vi "VIE.Module.Queued Message Handler.dqClass_ObjectReferenceToQueue.vi"(1 "reference":T1) -> (21 "queue":refnum<queue>)   [LabVIEW 2010, in "VIE.Module.Queued Message Handler.QueuedMessageHandler.dqGOOPClass.lvlib"]
doc: "Converts a dqGOOP object refnum to a queue refnum"
uses:
  VIE.Module.Queued Message Handler.QueuedMessageHandler.dqGOOPClass.lvlib
  VIE.Module.Queued Message Handler.dqClass_ObjectData.ctl
  VIE.Module.Queued Message Handler.dqClass_ObjectReference.ctl
panel:
  in  "queue (default)":refnum<queue>
  # "Copyright (C) 2004 DataAct Incorporated"
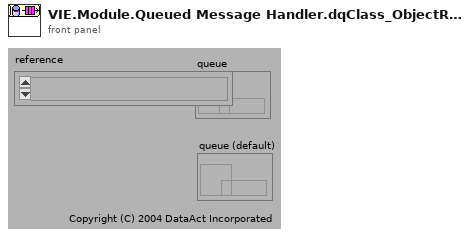
[diagram p1: front panel]
types:
  T1 = typedef "VIE.Module.Queued Message Handler.QueuedMessageHandler.dqGOOPClass.lvlib/VIE.Module.Queued Message Handler.dqClass_ObjectReference.ctl" = refnum<k1>
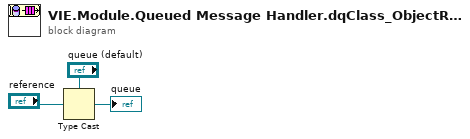
[diagram p0: block diagram]
diagram:
  n1 = Type Cast(type="queue (default)", x="reference") -> (*(type *) &x=→"queue":refnum<queue>)
